vi "APS set feeder point 2D ex.vi"(7 "LastFlag":i32, 8 "error in (no error)":errorcluster caption="错误输入（无错误）", 9 "Size":i32, 10 "PtArray":T1, 11 "GroupId":i32) -> (0 "error out":errorcluster caption="错误输出", 2 "PtArray out":T1, 3 "function return":i32)   [LabVIEW 2011, in "APS168.lvlib"]
doc: "I32 FNTYPE APS_set_feeder_point_2D_ex( I32 GroupId, PNT_DATA_2D_F64* PtArray, I32 Size, I32 LastFlag );"
uses:
  APS168.lvlib
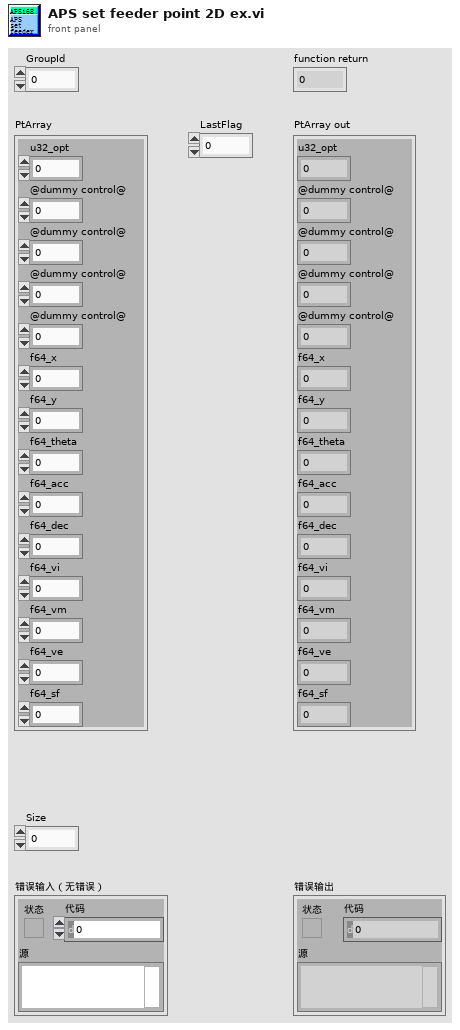
[diagram p1: front panel]
types:
  T1 = cluster{"u32_opt":u32, "@dummy control@":i8, "@dummy control@":i8, "@dummy control@":i8, "@dummy control@":i8, "f64_x":dbl, "f64_y":dbl, "f64_theta":dbl, "f64_acc":dbl, "f64_dec":dbl, "f64_vi":dbl, "f64_vm":dbl, "f64_ve":dbl, "f64_sf":dbl}
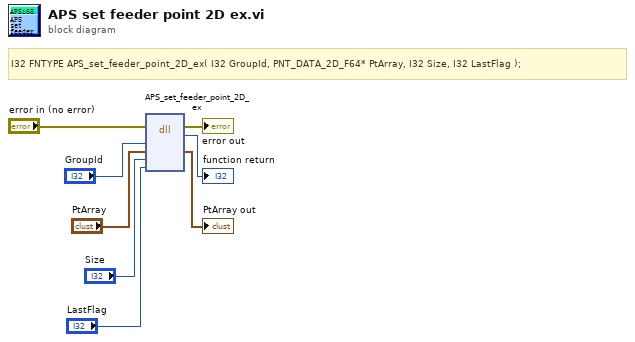
[diagram p0: block diagram]
diagram:
  # "I32 FNTYPE APS_set_feeder_point_2D_ex( I32 GroupId, PNT_DATA_2D_F64* PtArray, I32 Size, I32 LastFlag );"
  n1 = dll-call lib="PTH1Labs E软件ADLINK 204CAPS_1_7_1_LIB line 连续运动204APS168.*" fn="APS_set_feeder_point_2D_ex"(error in="error in (no error)", "GroupId"="GroupId", "PtArray"="PtArray", "Size"="Size", "LastFlag"="LastFlag") -> (error out=→"error out":errorcluster, →"function return":i32, "PtArray"=→"PtArray out":T1)  [unwired: 5 in, 1 out]
